vi "MM9.InitAFGs.vi"(0 "i ref in":refnum<vi>, 2 "InitObjs":string[](array[string]), 3 "ms timeout (10000)":i32=10000, 5 "error in (no error)":errorcluster) -> (14 "i ref out":refnum<vi>, 16 "InitObjs out":string[](array[string]), 17 "timed out":bool, 19 "error out":errorcluster)   [LabVIEW 2014, in "MM9.lvlib"]
doc: "This method loads all AFGs."
uses:
  MM9.lvlib
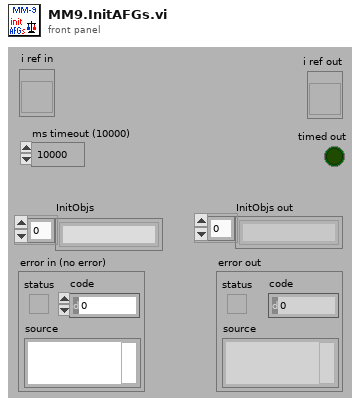
[diagram p1: front panel]
types:
  T1 = typedef "MM9.lvlib/MM9.i attribute.ctl" = cluster{"UsedObjs":string[], "ActScanStep":i32[], "AbortRequest":bool, "StopRequest":bool, "# cycles":i32, "Connected":bool, "MMStatus":T2, "# data":i32, "DIMServices":cluster{"MM6StatusString":string, "MM6StatusID":i32, "discArchiver":string, "discArchiverID":i32, "eventBuilder":string, "eventBuilderID":i32, "GUIIDString":string, "GUIIDStringID":i32}, "dataFile":string, "PGRunning":T3, "ConfigData":T4, "ExtraDataSets":T19}
  T2 = typedef "MM9.lvlib/MM9.status.ctl" = enum16{"loaded", "load_error", "config", "config_error", "init", "init_error", "data_reset", "data_reset_error", "running", "start_error", "run_error", "abort_requested", "aborted", "stop_requested", "stopped", "stop_error", "Connected", "NOTConnected"}
  T3 = typedef "PPG_ABC.lvlib/PPG_ABC.PG_Running.ctl" = i32
  T4 = typedef "LEBITDefs9.lvlib/LEBITDefs.ConfigData.ctl" = cluster{"GenConfig":T5, "Configs":T7[]}
  T5 = typedef "LEBITDefs9.lvlib/LEBITDefs.GenConfig.ctl" = cluster{"Mode":i32, "Logs":T6[]}
  T6 = typedef "LEBITDefs9.lvlib/LEBITDefs.Log.ctl" = cluster{"Name":string, "FctName":string, "Special":string}
  T7 = typedef "LEBITDefs9.lvlib/LEBITDefs.OneConfig.ctl" = cluster{"MCA":T8, "Timing":T9, "Scans":T12[], "FreqDevs":T13[], "CleanDev":T14, "NrCycles":i32, "Specials":T16[], "Delays":T17[], "DAC":T18}
  T8 = typedef "LEBITDefs9.lvlib/LEBITDefs.MCA.ctl" = cluster{"Name":string, "Address":string, "NrChannels":i32, "Gate":i32, "NrPipse":i32, "AcqDelay":i32}
  T9 = typedef "LEBITDefs9.lvlib/LEBITDefs.Timing.ctl" = cluster{"TimeTables":cluster{"TimeTable":T10}[], "Memories":T11[], "ScanX":string, "ScanY":string}
  T10 = typedef "LEBITDefs9.lvlib/LEBITDefs.Timetable.ctl" = dbl[]
  T11 = typedef "LEBITDefs9.lvlib/LEBITDefs.Memory.ctl" = cluster{"Device":string, "ExtTrig":bool, "TT2Use":i32, "PatternTable":string[]}
  T12 = typedef "LEBITDefs9.lvlib/LEBITDefs.ScanDev.ctl" = cluster{"Name":string, "FctName":string, "Values":dbl[], "NrScanVals":i32, "Special":string}
  T13 = typedef "LEBITDefs9.lvlib/LEBITDefs.FreqDev.ctl" = cluster{"Name":string, "Amp":dbl, "CenterFreq":dbl, "Time":dbl}
  T14 = typedef "LEBITDefs9.lvlib/LEBITDefs.CleanDev.ctl" = cluster{"Name":string, "CleanData":T15[]}
  T15 = typedef "LEBITDefs9.lvlib/LEBITDefs.CleanDataType.ctl" = cluster{"Amp":dbl, "Center":dbl, "Plus":dbl, "Minus":dbl, "Time":dbl}
  T16 = typedef "LEBITDefs9.lvlib/LEBITDefs.Special.ctl" = cluster{"Name":string, "FctName":string, "VerySpecial":string, "Data":dbl}
  T17 = typedef "LEBITDefs9.lvlib/LEBITDefs.Delay.ctl" = cluster{"Name":string, "Delay":dbl}
  T18 = typedef "LEBITDefs9.lvlib/LEBITDefs.DAC.ctl" = cluster{"Name":string, "Step1":i32, "Step2":i32}
  T19 = typedef "LEBITDefs9.lvlib/LEBITDefs.ExtraData.ctl" = cluster{"Ions":cluster{"ExcitIonMass":string, "ExcitIonCharge":i32, "CleanIons":cluster{"CleanIonMass":string, "CleanIonCharge":i32}[]}, "TimingDescription":cluster{"TimeTableDescription":cluster{"Times":string[]}[], "PatternTableDescription":cluster{"Pattern":string[]}[]}, "ScanUnits":string[]}[]
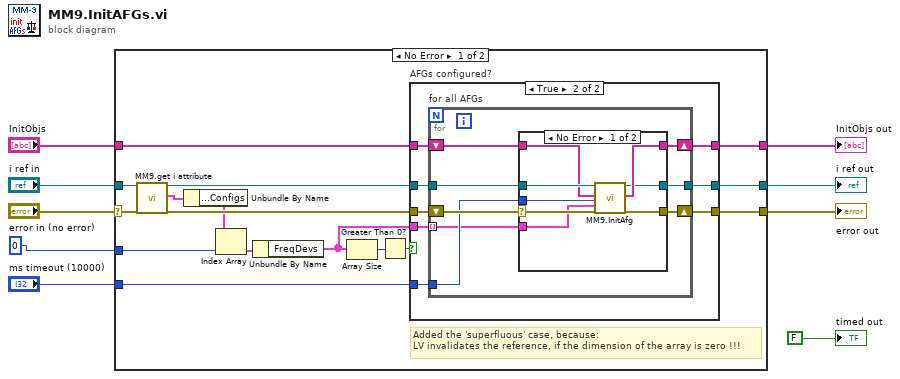
[diagram p0: block diagram]
diagram:
  n1 = case shown="No Error" "error in (no error)" {
    selector: "error in (no error)" -> [w24 w57]
    tunnel: "i ref in" -> [w25 w58]
    tunnel: "InitObjs" -> [w21 w56]
    tunnel: [w20 w57] -> w5
    tunnel: [w19 w58] -> w4
    tunnel: "ms timeout (10000)" -> [w18 _]
    tunnel: [w17 w56] -> w2
    tunnel: 0 ("index") -> [w11 _]
    frame No Error {
      # "Added the 'superfluous' case, because:\nLV invalidates the reference, if the dimension of the array is zero !!!"
      n2 = call "MM9.get i attribute.vi"("i ref in"=w25, "error in (no error)"=w24) -> ("i ref out"=w22:refnum<vi>, "i attribute"=w14:T1, "error out"=w23:errorcluster)  [unwired: 15 in]
      n3 = Unbundle By Name(w14) -> ("ConfigData.Configs"=w13:T7[])
      n4 = Index Array(array=w13, index=w11) -> (element=w12:T7)
      n5 = Unbundle By Name(w12) -> ("FreqDevs"=w10:T13[])
      n6 = Array Size(array=w10) -> (size(s)=w16:i32)
      n7 = Greater Than 0?(x=w16) -> (x > 0?=w15:bool)
      n8 = case "AFGs configured?" shown="True" w15 {
        tunnel: w23 -> [w27 w36]
        tunnel: w22 -> [w28 w35]
        tunnel: w21 -> [w26 w34]
        tunnel: [w27 w33] -> w20
        tunnel: [w28 w32] -> w19
        tunnel: w18 -> [_ w31]
        tunnel: [w26 w30] -> w17
        tunnel: w10 -> [_ w29]
        frame False {
        }
        frame True {
          n9 = for "for all AFGs" {
            shift-right: [w40] -> w33
            shift-left: w36 -> [w44]
            tunnel: w35 -> [w43]
            shift-right: [w41] -> w30
            shift-left: w34 -> [w42]
            tunnel: [w39] -> w32
            tunnel: w31 -> [w38]
            tunnel: w29 -> [w37] mode=indexing
            n10 = case shown="No Error" w44 {
              selector: w44 -> [w51 w54]
              tunnel: w43 -> [w52 w53]
              tunnel: w42 -> [w50 w55]
              tunnel: [w49 w55] -> w41
              tunnel: [w48 w54] -> w40
              tunnel: [w47 w53] -> w39
              tunnel: w38 -> [w46 _]
              tunnel: w37 -> [w45 _]
              frame No Error {
                n11 = call "MM9.InitAfg.vi"("i ref in"=w52, "InitObjs"=w50, "ms timeout (10000)"=w46, "FreqDev"=w45, "error in (no error)"=w51) -> ("i ref out"=w47:refnum<vi>, "InitObjs out"=w49:string[], "error out"=w48:errorcluster)  [unwired: 11 in, 1 out]
              }
              frame Error {
              }
            }
          }
        }
      }
    }
    frame Error {
    }
  }
  "error out" <- w5
  "i ref out" <- w4
  "InitObjs out" <- w2
  "timed out" <- FALSE ("timed out")
